vi "StallDetection.vi"(9 "Required Stall Time (s)":dbl, 10 "Stall Current":dbl, 11 "Current In":dbl) -> (3 "Stalled?":bool)   [LabVIEW 2017]
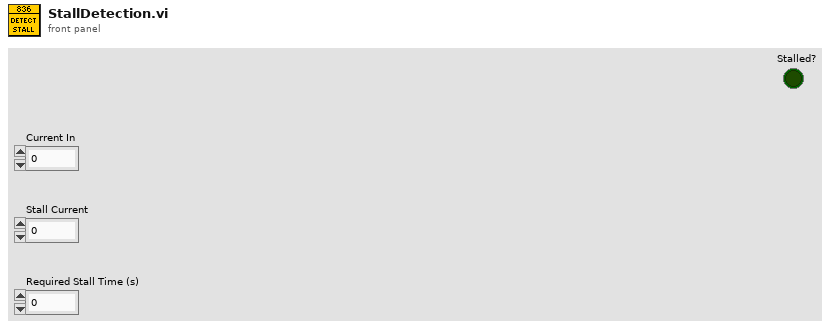
[diagram p1: front panel]
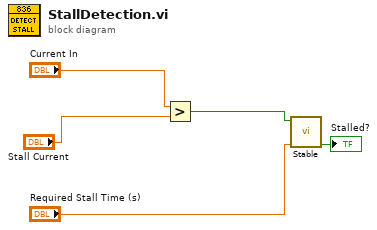
[diagram p0: block diagram]
diagram:
  n1 = Greater?(x="Current In", y="Stall Current") -> (0:w3:bool)
  n2 = call <userlib>:"Stable.vi"("Eval Period (sec)"="Required Stall Time (s)", "Signal Input"=w3) -> ("Stable"=→"Stalled?":bool)  [unwired: 9 in]
